vi "DAQ2ANA Data Interface.vi"(8 "error in":errorcluster, 9 "UsedChList[]":T1(array[cluster]), 11 "Tree Ref":refnum<vi>) -> (0 "error out":errorcluster, 1 "VariList":cluster{"Tag[]":string[], "Name[]":string[]})   [LabVIEW 2016]
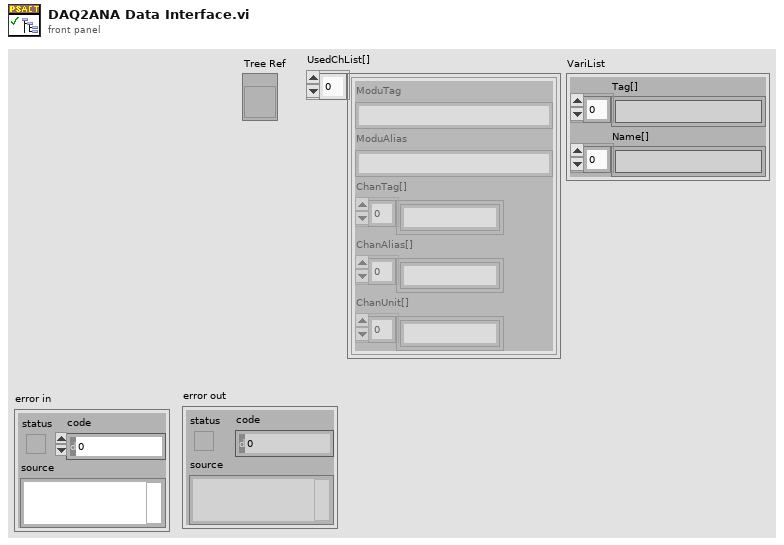
[diagram p1: front panel]
types:
  T1 = cluster{"ModuTag":string, "ModuAlias":string, "ChanTag[]":string[], "ChanAlias[]":string[], "ChanUnit[]":string[]}[]
  T2 = cluster{"Left Cell String":string, "Child Text":string[], "Child Tag":string, "Item Indent":i32, "Child Only?":bool, "Glyph Index":i32}
  T3 = cluster{"Left Cell String":string, "Child Text":string[], "Child Tag":string, "Item Indent":i32, "Child Only?":bool, "Glyph Index":i32}[]
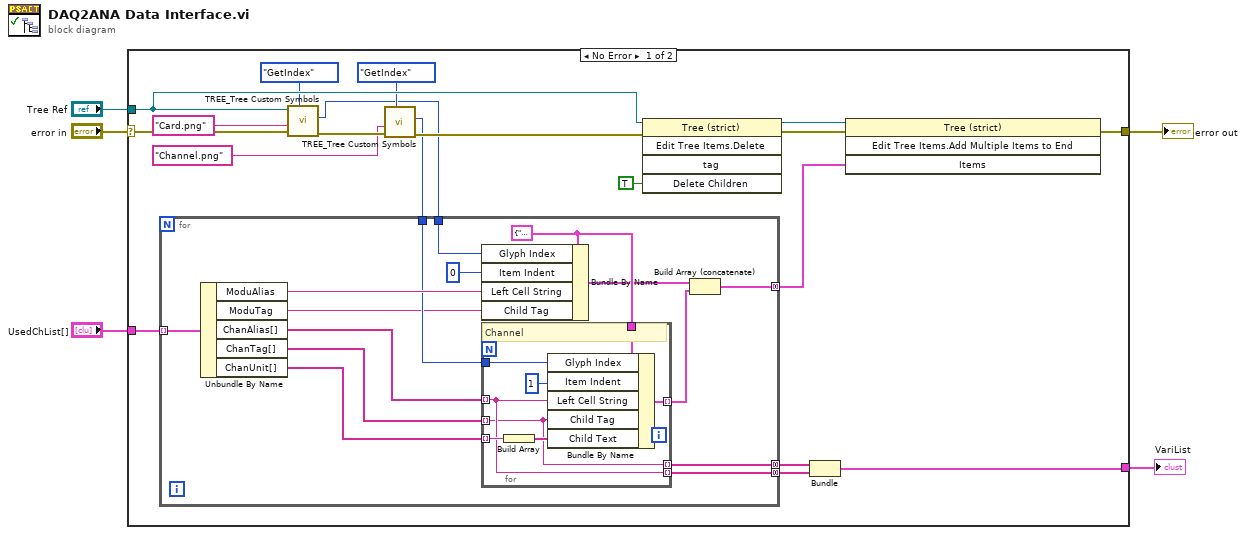
[diagram p0: block diagram]
diagram:
  n1 = case shown="No Error" "error in" {
    selector: "error in" -> [w20 w48]
    tunnel: [w21 w48] -> w5
    tunnel: "Tree Ref" -> [w19 _]
    tunnel: "UsedChList[]" -> [w9 _]
    tunnel: [w6 _] -> w1
    frame No Error {
      n2 = call "TREE_Tree Custom Symbols.vi"("Operation"=enum16{"Register", "GetIndex"}."GetIndex", "error in"=w20, "PicName"="Card.png", "tree refnum"=w19) -> ("error out"=w15:errorcluster, "PicIndex"=w12:i32)  [unwired: 6 in]
      n3 = call "TREE_Tree Custom Symbols.vi"("Operation"=enum16{"Register", "GetIndex"}."GetIndex", "error in"=w15, "PicName"="Channel.png") -> ("error out"=w14:errorcluster, "PicIndex"=w13:i32)  [unwired: 7 in]
      n4 = for {
        tunnel: w9 -> [w39] mode=indexing
        tunnel: [w33] -> w10 mode=concatenating
        tunnel: [w32] -> w8 mode=concatenating
        tunnel: [w31] -> w7 mode=concatenating
        tunnel: w13 -> [w29]
        tunnel: w12 -> [w30]
        w36 = T2 {"Left Cell String"="", "Child Text"=[], "Child Tag"="", "Item Indent"=0, "Child Only?"=FALSE, "Glyph Index"=0} ("Item")
        n5 = Unbundle By Name(w39) -> ("ModuAlias"=w38:string, "ModuTag"=w28:string, "ChanAlias[]"=w27:string[], "ChanTag[]"=w26:string[], "ChanUnit[]"=w25:string[])
        n6 = Bundle By Name(cluster=w36, "Glyph Index"=w30, "Item Indent"=0, "Left Cell String"=w38, "Child Tag"=w28) -> (w35:T2)
        n7 = for {
          tunnel: w27 -> [w42] mode=indexing
          tunnel: w36 -> [w47]
          tunnel: [w46] -> w34 mode=indexing
          tunnel: w26 -> [w40] mode=indexing
          tunnel: w25 -> [w44] mode=indexing
          tunnel: [w40] -> w32 mode=indexing
          tunnel: [w42] -> w31 mode=indexing
          tunnel: w29 -> [w41]
          # "Channel"
          n8 = Build Array(w44) -> (w45:string[])
          n9 = Bundle By Name(cluster=w47, "Glyph Index"=w41, "Item Indent"=1, "Left Cell String"=w42, "Child Tag"=w40, "Child Text"=w45) -> (w46:T2)
        }
        n10 = Build Array (concatenate)(w35, w34) -> (w33:T3)
      }
      n11 = invoke class="Tree (strict)" method="Edit Tree Items.Delete"(reference=w19, error in=w14, "Delete Children"=TRUE ("Delete Children?")) -> (reference out=w23:refnum<vi>, error out=w22:errorcluster)  [unwired: 2 in, 3 out]
      n12 = Bundle(w8, w7) -> (w6:cluster{string[], string[]})  [unwired: 1 in]
      n13 = invoke class="Tree (strict)" method="Edit Tree Items.Add Multiple Items to End"(reference=w23, error in=w22, "Items"=w10) -> (error out=w21:errorcluster)  [unwired: 1 in, 3 out]
    }
    frame Error {
    }
  }
  "error out" <- w5
  "VariList" <- w1
